vi "8X(json).vi"(0 "xml path":path=path "D:/wmgxml.xml", 1 "type":T4(ring)=enum."QSFP28", 5 "txtPath":path, 7 "singleItemInfo":T3[](array[typedef]), 9 "xml_detail":T1, 11 "TDD":T2) -> ()   [LabVIEW 2011]
uses:
  dataType/sSpec.ctl
  dataType/TDD.ctl
  dataType/xml_detail.ctl
panel:
  out "cycle item names":string[](array[string])
  out "midVar_time":string[](array[string])
  out "cycle items":string[](array[string])
  out "Terminat Points":dbl[](array[numeric])
  out "TDD spec cable":string
  out "TDD spec terminal":string
  out "Cable Points":dbl[](array[numeric])
  out "TestResult":string
  out "input_array_time":string[](array[string])
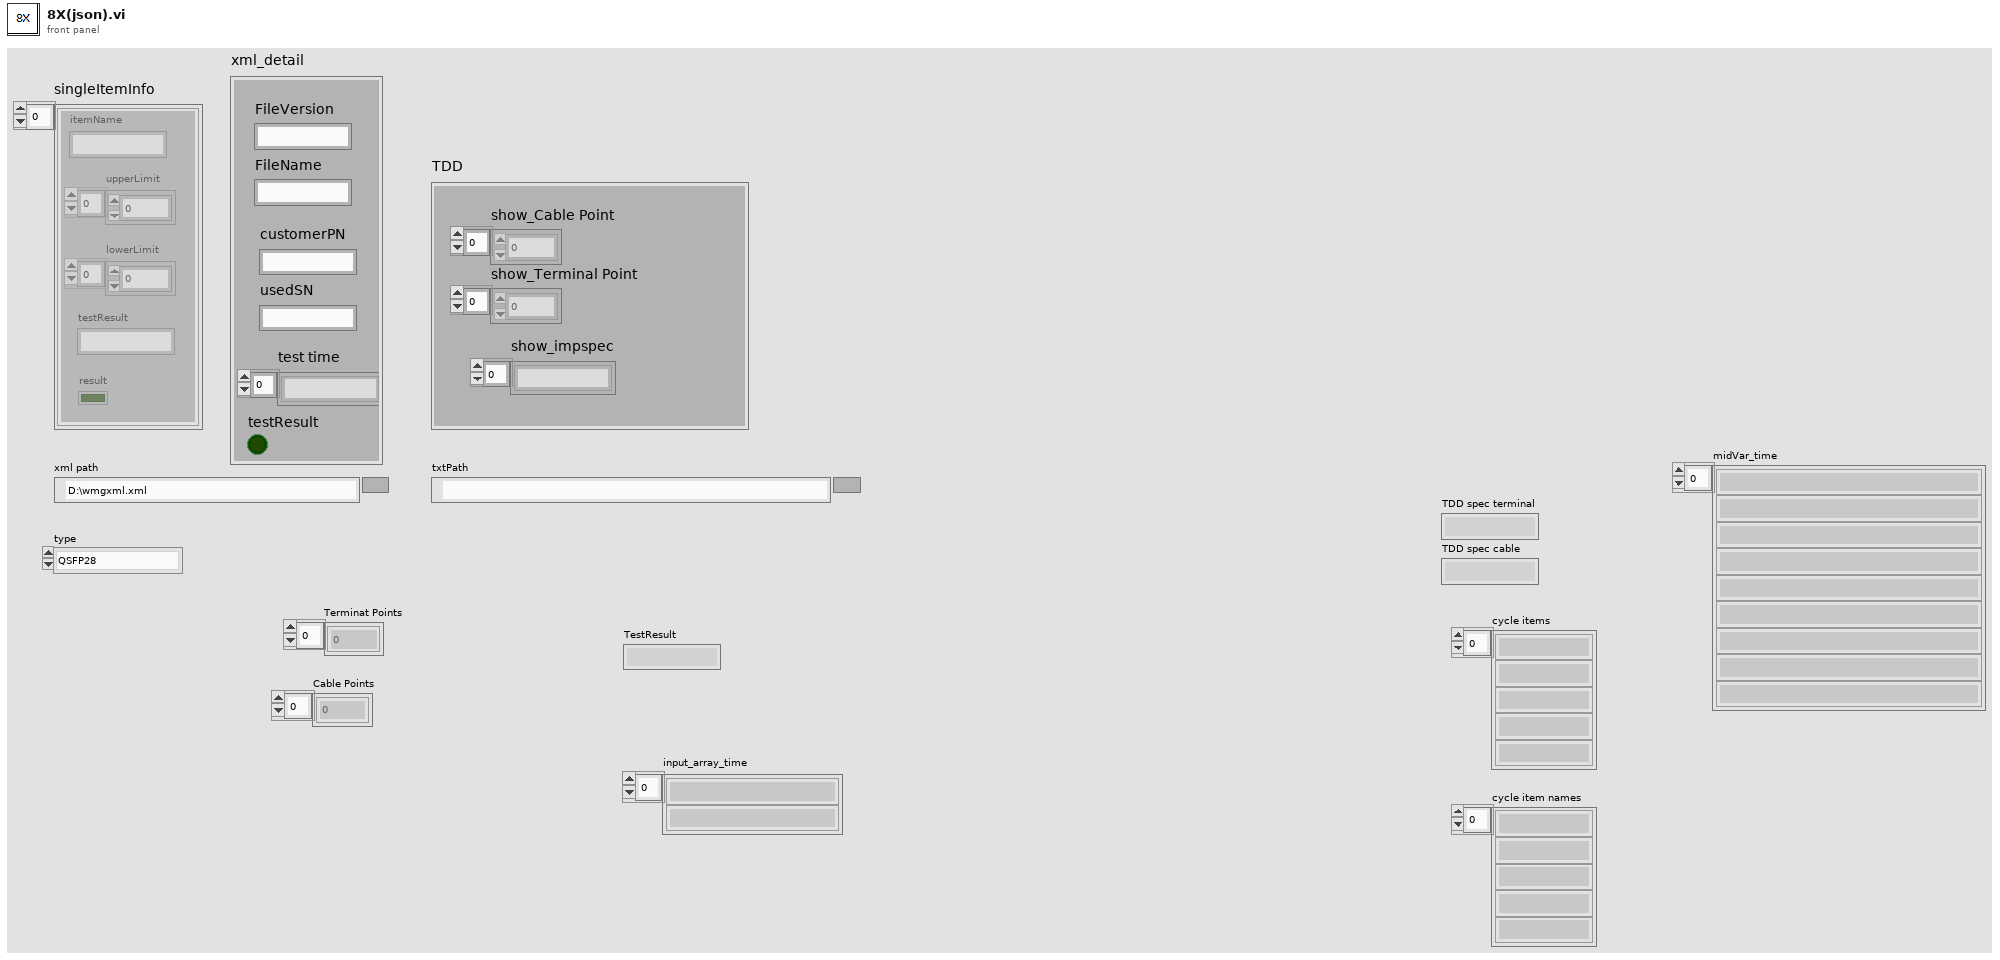
[diagram p1: front panel]
types:
  T1 = typedef "xml_detail.ctl" = cluster{"FileVersion":string, "FileName":string, "customerPN":string, "usedSN":string, "test time":string[], "testResult":bool}
  T2 = typedef "TDD.ctl" = cluster{"show_Cable Point":dbl[], "show_Terminal Point":dbl[], "show_impspec":string[]}
  T3 = typedef "sSpec.ctl" = cluster{"itemName":string, "upperLimit":dbl[], "lowerLimit":dbl[], "testResult":string, "result":bool}
  T4 = enum16{"MINI SAS HD 4X", "MINI SAS 4X", "SFP28", "QSFP28", "SFP+", "SLIM"}
  T5 = enum16{"open", "replace", "create", "open or create", "replace or create", "replace or create with confirmation"}
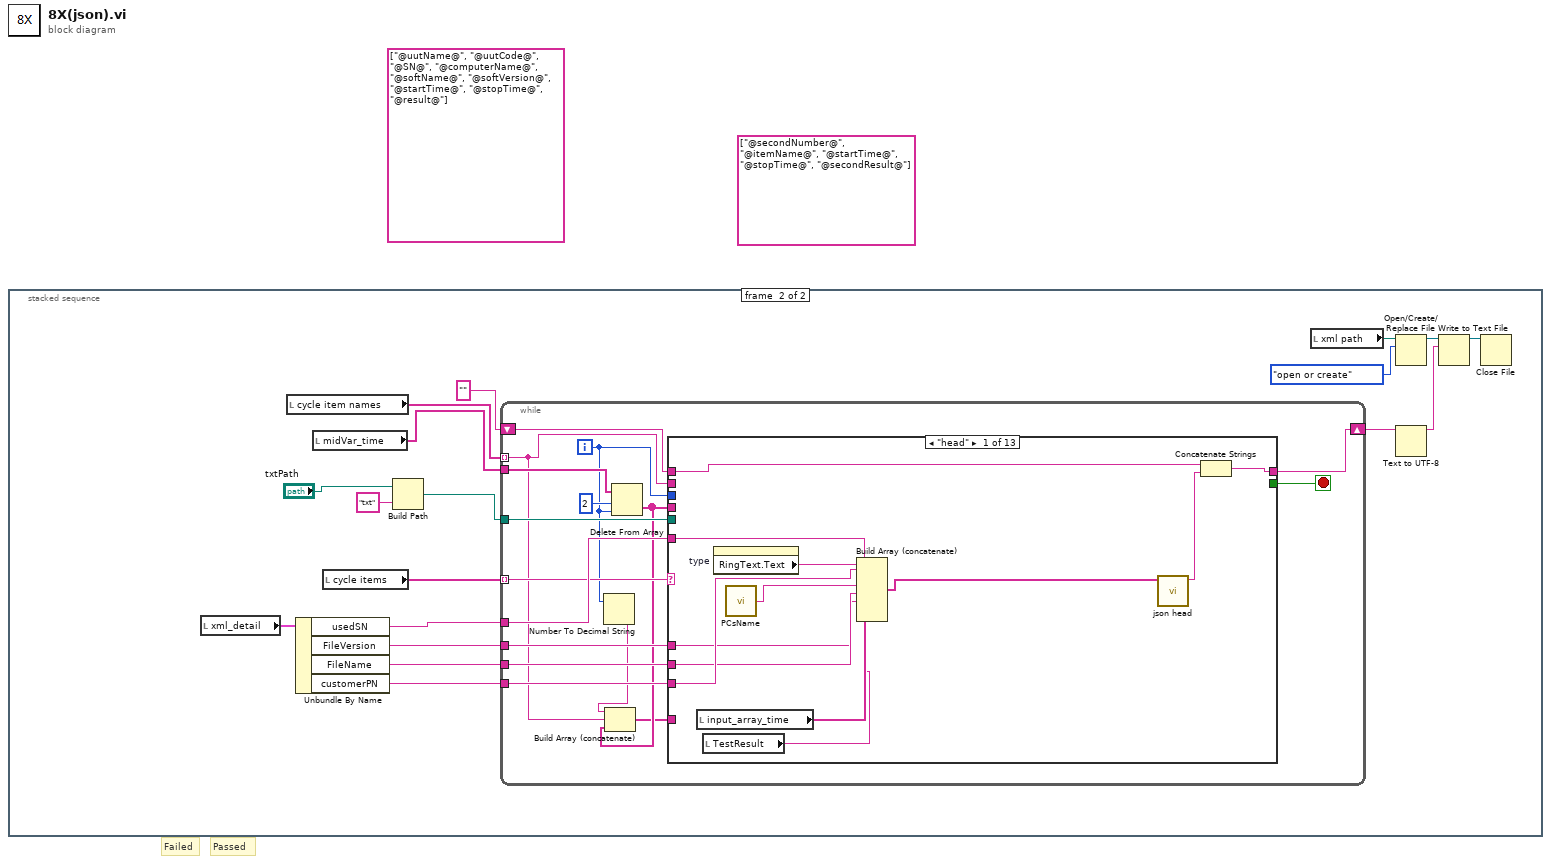
[diagram p0: block diagram]
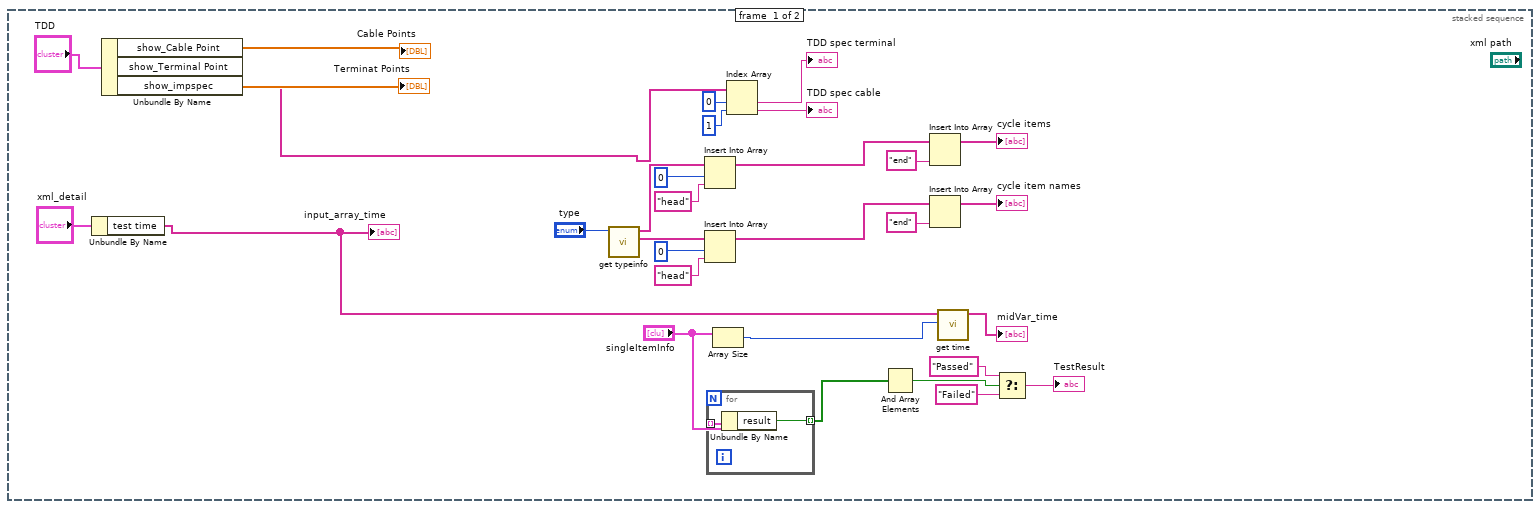
[diagram p2: hidden frame]
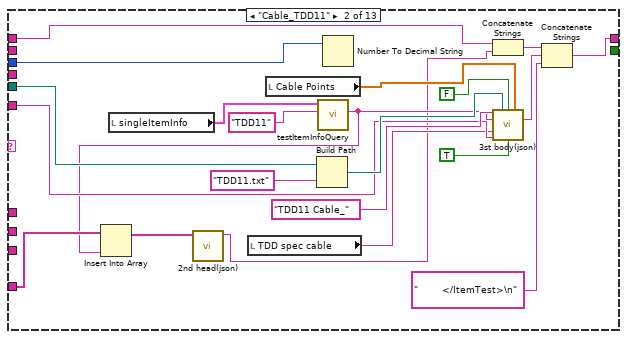
[diagram p3: hidden frame]
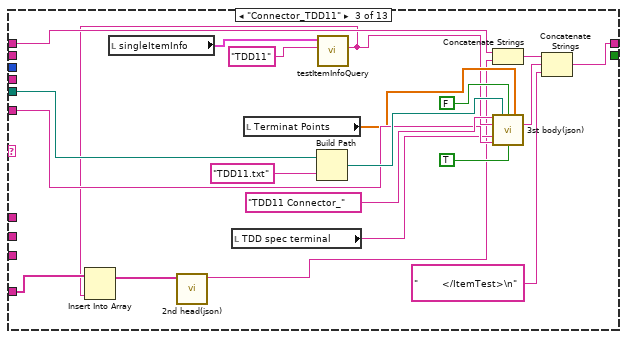
[diagram p4: hidden frame]
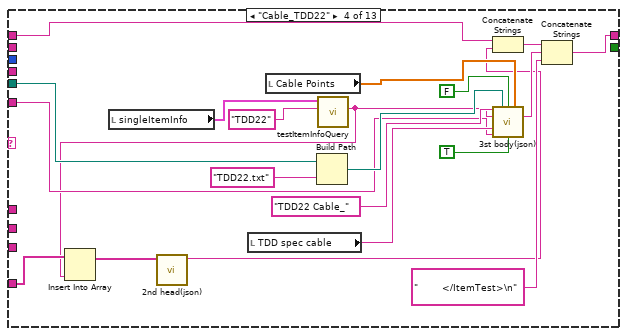
[diagram p5: hidden frame]
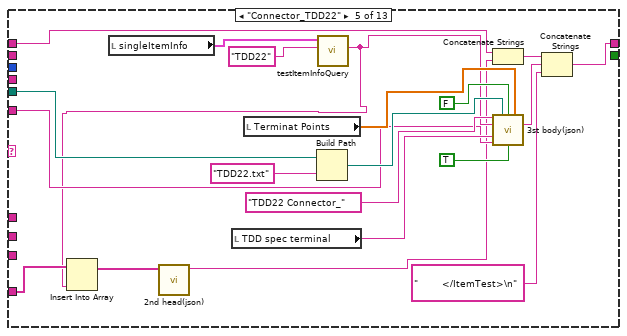
[diagram p6: hidden frame]
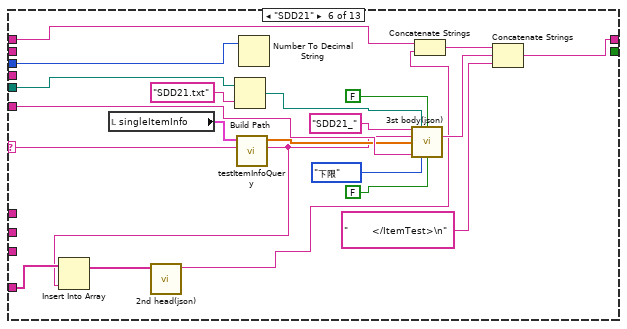
[diagram p7: hidden frame]
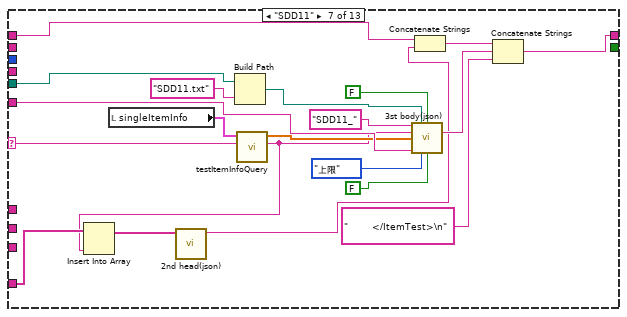
[diagram p8: hidden frame]
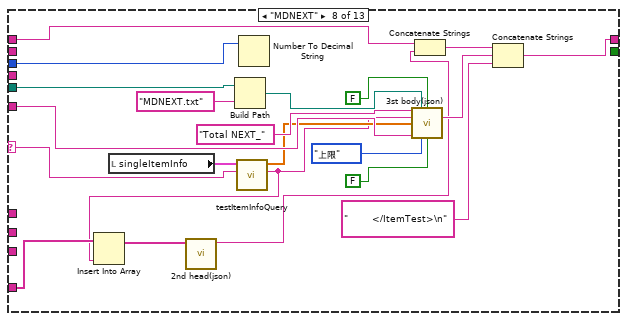
[diagram p9: hidden frame]
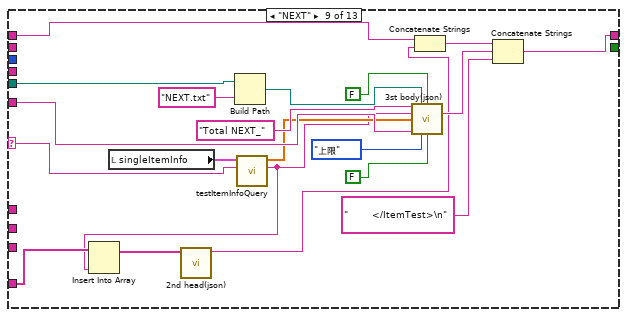
[diagram p10: hidden frame]
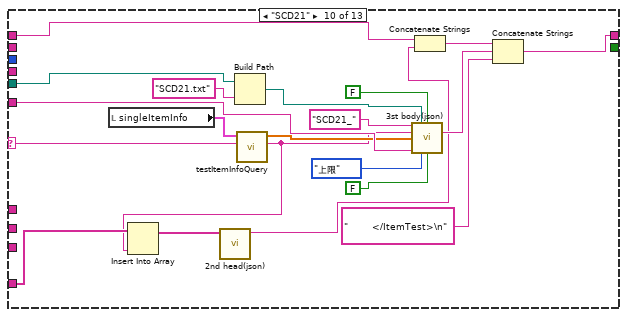
[diagram p11: hidden frame]
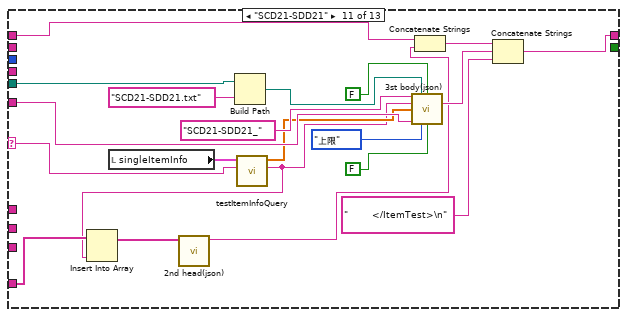
[diagram p12: hidden frame]
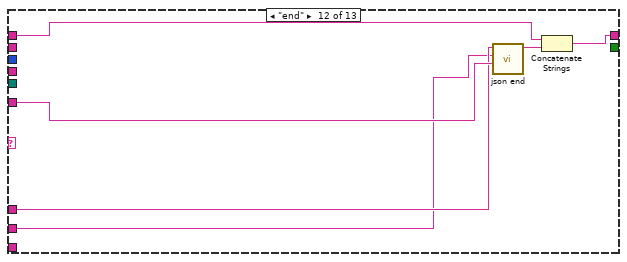
[diagram p13: hidden frame]
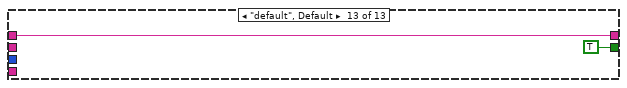
[diagram p14: hidden frame]
diagram:
  (unwired) string[] ["@uutName@", "@uutCode@", "@SN@", "@computerName@", "@softName@", "@softVersion@", "@startTime@", "@stopTime@", "@result@"]
  (unwired) string[] ["@secondNumber@", "@itemName@", "@startTime@", "@stopTime@", "@secondResult@"]
  # "Failed"
  # "Passed"
  n1 = stacked-sequence {
    frame #0 {
      n2 = Unbundle By Name("xml_detail") -> ("test time"=w1:string[])
      "input_array_time" <- w1
      n3 = Unbundle By Name("TDD") -> ("show_Cable Point"=→"Cable Points":dbl[], "show_Terminal Point"=→"Terminat Points":dbl[], "show_impspec"=w3:string[])
      n4 = call "get typeinfo.vi"("type"="type") -> ("second item names"=w15:string[], "test items"=w16:string[])  [unwired: 9 in]
      n5 = Insert Into Array(array=w16, index=0 ("索引"), new element="head" ("新元素/子数组")) -> (w25:string[])
      n6 = Insert Into Array(array=w15, index=0 ("索引"), new element="head" ("新元素/子数组")) -> (w19:string[])
      n7 = for {
        tunnel: "singleItemInfo" -> [w33] mode=indexing
        tunnel: [w32] -> w7 mode=indexing
        n8 = Unbundle By Name(w33) -> ("result"=w32:bool)
      }
      n9 = Array Size(array="singleItemInfo") -> (size(s)=w9:i32)
      n10 = Index Array(array=w3, index #1=0 ("索引"), index #2=1 ("索引")) -> (element #1=→"TDD spec terminal":string, element #2=→"TDD spec cable":string)
      n11 = And Array Elements(Boolean array=w7) -> (logical AND=w11:bool)
      n12 = Insert Into Array(array=w25, new element="end" ("新元素/子数组")) -> (→"cycle items":string[])  [unwired: 1 in]
      n13 = Insert Into Array(array=w19, new element="end" ("新元素/子数组")) -> (→"cycle item names":string[])  [unwired: 1 in]
      n14 = call "get time.vi"("item count"=w9, "input_array_time"=w1) -> ("midVar_time"=→"midVar_time":string[])  [unwired: 9 in]
      n15 = Select(t="Passed", s=w11, f="Failed") -> (s? t:f=→"TestResult":string)
    }
    frame #1 {
      n16 = local read "xml_detail"() -> (w38:T1)
      n17 = local read "cycle item names"() -> (w42:string[])
      n18 = Unbundle By Name(w38) -> ("usedSN"=w37:string, "FileVersion"=w36:string, "FileName"=w35:string, "customerPN"=w34:string)
      n19 = local read "midVar_time"() -> (w43:string[])
      n20 = local read "cycle items"() -> (w50:string[])
      n21 = Build Path(base path="txtPath", name or relative path="txt" ("名称或相对路径")) -> (appended path=w39:path)
      n22 = while {
        tunnel: w50 -> [w62] mode=indexing
        shift-right: [w66] -> w45
        shift-left: "" -> [w67]
        tunnel: w39 -> [w65]
        tunnel: w37 -> [w64]
        tunnel: w43 -> [w61]
        tunnel: w42 -> [w54] mode=indexing
        tunnel: w36 -> [w59]
        tunnel: w35 -> [w58]
        tunnel: w34 -> [w57]
        i -> [w56]
        stop <- w63 stop-if-true
        n23 = Number To Decimal String(number=w56) -> (decimal integer string=w55:string)  [unwired: 1 in]
        n24 = Delete From Array(array=w61, length=2 ("长度"), index=w56) -> (deleted portion=w53:string[])  [unwired: 1 out]
        n25 = Build Array (concatenate)(w55, w54, w53) -> (w52:string[])
        n26 = case shown="\"head\"" w62 {
          selector: w62 -> [_ _ _ _ _ w165 w186 w206 w227 w247 w267 _ _]
          tunnel: w67 -> [w79 w99 w120 w140 w160 w180 w201 w221 w242 w262 w282 w287 w290]
          tunnel: [w78 w96 w117 w137 w157 w177 w198 w218 w239 w259 w279 w286 w290] -> w66
          tunnel: w56 -> [_ w100 _ _ _ w181 _ w222 _ _ _ _ _]
          tunnel: w65 -> [_ w93 w114 w134 w154 w174 w195 w215 w236 w256 w276 _ _]
          tunnel: w64 -> [w74 w88 w109 w127 w147 w169 w190 w210 w231 w251 w271 w285 _]
          tunnel: [_ _ _ _ _ _ _ _ _ _ _ _ TRUE] -> w63
          tunnel: w53 -> [_ _ _ _ _ _ _ _ _ _ _ _ _]
          tunnel: w54 -> [_ _ _ _ _ _ _ _ _ _ _ _ _]
          tunnel: w59 -> [w71 _ _ _ _ _ _ _ _ _ _ w284 _]
          tunnel: w58 -> [w72 _ _ _ _ _ _ _ _ _ _ w283 _]
          tunnel: w57 -> [w75 _ _ _ _ _ _ _ _ _ _ _ _]
          tunnel: w52 -> [_ w83 w103 w123 w143 w163 w184 w204 w225 w245 w265 _ _]
          frame "head" {
            n27 = local read "input_array_time"() -> (w70:string[])
            n28 = local read "TestResult"() -> (w69:string)
            n29 = property on="type" class="Enum (严格)"() -> ("RingText.Text"=w76:string)  [unwired: 2 in, 2 out]
            n30 = call "PCsName.vi"() -> ("Computer Name"=w73:string)
            n31 = Build Array (concatenate)(w76, w75, w74, w73, w72, w71, w70, w69) -> (w68:string[])
            n32 = call "json head.vi"("information"=w68) -> ("midVar_Content"=w77:string)  [unwired: 10 in]
            n33 = Concatenate Strings(w79, w77) -> (w78:string)
          }
          frame "Cable_TDD11" {
            n34 = local read "singleItemInfo"() -> (w85:T3[])
            n35 = local read "TDD spec cable"() -> (w87:string)
            n36 = local read "Cable Points"() -> (w86:dbl[])
            n37 = Build Path(base path=w93, name or relative path="TDD11.txt" ("名称或相对路径")) -> (appended path=w91:path)
            n38 = call "testItemInfoQuery.vi"("testItem"="TDD11" ("test item"), "singleItemInfo"=w85) -> ("testResult"=w81:string)  [unwired: 8 in, 1 out]
            n39 = Insert Into Array(array=w83, new element=w81) -> (w82:string[])  [unwired: 1 in]
            n40 = call "2nd head(json).vi"("value"=w82) -> ("midVar_Content"=w80:string)  [unwired: 10 in]
            n41 = Number To Decimal String(number=w100) -> ()  [unwired: 1 in, 1 out]
            n42 = Concatenate Strings(w99, w80) -> (w97:string)
            n43 = call "3st body(json).vi"("third test item name"="TDD11 Cable_", "file path (dialog if empty)"=w91, "ABS?"=FALSE, "Points"=w86, "second result"=w81, "TDD spec"=w87, "SN"=w88, "TDD?"=TRUE) -> ("OutPutXml"=w95:string)  [unwired: 7 in]
            n44 = Concatenate Strings(w97, w95, "        </ItemTest>\n") -> (w96:string)
          }
          frame "Connector_TDD11" {
            n45 = local read "singleItemInfo"() -> (w106:T3[])
            n46 = local read "TDD spec terminal"() -> (w107:string)
            n47 = local read "Terminat Points"() -> (w108:dbl[])
            n48 = Build Path(base path=w114, name or relative path="TDD11.txt" ("名称或相对路径")) -> (appended path=w112:path)
            n49 = call "testItemInfoQuery.vi"("testItem"="TDD11" ("test item"), "singleItemInfo"=w106) -> ("testResult"=w102:string)  [unwired: 8 in, 1 out]
            n50 = Insert Into Array(array=w103, new element=w102) -> (w104:string[])  [unwired: 1 in]
            n51 = call "2nd head(json).vi"("value"=w104) -> ("midVar_Content"=w101:string)  [unwired: 10 in]
            n52 = Concatenate Strings(w120, w101) -> (w118:string)
            n53 = call "3st body(json).vi"("third test item name"="TDD11 Connector_", "file path (dialog if empty)"=w112, "ABS?"=FALSE, "Points"=w108, "second result"=w102, "TDD spec"=w107, "SN"=w109, "TDD?"=TRUE) -> ("OutPutXml"=w116:string)  [unwired: 7 in]
            n54 = Concatenate Strings(w118, w116, "        </ItemTest>\n") -> (w117:string)
          }
          frame "Cable_TDD22" {
            n55 = local read "singleItemInfo"() -> (w126:T3[])
            n56 = local read "TDD spec cable"() -> (w128:string)
            n57 = local read "Cable Points"() -> (w129:dbl[])
            n58 = Build Path(base path=w134, name or relative path="TDD22.txt" ("名称或相对路径")) -> (appended path=w132:path)
            n59 = call "testItemInfoQuery.vi"("testItem"="TDD22" ("test item"), "singleItemInfo"=w126) -> ("testResult"=w122:string)  [unwired: 8 in, 1 out]
            n60 = Insert Into Array(array=w123, new element=w122) -> (w124:string[])  [unwired: 1 in]
            n61 = call "2nd head(json).vi"("value"=w124) -> ("midVar_Content"=w121:string)  [unwired: 10 in]
            n62 = Concatenate Strings(w140, w121) -> (w138:string)
            n63 = call "3st body(json).vi"("third test item name"="TDD22 Cable_", "file path (dialog if empty)"=w132, "ABS?"=FALSE, "Points"=w129, "second result"=w122, "TDD spec"=w128, "SN"=w127, "TDD?"=TRUE) -> ("OutPutXml"=w136:string)  [unwired: 7 in]
            n64 = Concatenate Strings(w138, w136, "        </ItemTest>\n") -> (w137:string)
          }
          frame "Connector_TDD22" {
            n65 = local read "singleItemInfo"() -> (w146:T3[])
            n66 = local read "TDD spec terminal"() -> (w148:string)
            n67 = local read "Terminat Points"() -> (w149:dbl[])
            n68 = Build Path(base path=w154, name or relative path="TDD22.txt" ("名称或相对路径")) -> (appended path=w152:path)
            n69 = call "testItemInfoQuery.vi"("testItem"="TDD22" ("test item"), "singleItemInfo"=w146) -> ("testResult"=w142:string)  [unwired: 8 in, 1 out]
            n70 = Insert Into Array(array=w143, new element=w142) -> (w144:string[])  [unwired: 1 in]
            n71 = call "2nd head(json).vi"("value"=w144) -> ("midVar_Content"=w141:string)  [unwired: 10 in]
            n72 = Concatenate Strings(w160, w141) -> (w158:string)
            n73 = call "3st body(json).vi"("third test item name"="TDD22 Connector_", "file path (dialog if empty)"=w152, "ABS?"=FALSE, "Points"=w149, "second result"=w142, "TDD spec"=w148, "SN"=w147, "TDD?"=TRUE) -> ("OutPutXml"=w156:string)  [unwired: 7 in]
            n74 = Concatenate Strings(w158, w156, "        </ItemTest>\n") -> (w157:string)
          }
          frame "SDD21" {
            n75 = local read "singleItemInfo"() -> (w167:T3[])
            n76 = Build Path(base path=w174, name or relative path="SDD21.txt" ("名称或相对路径")) -> (appended path=w172:path)
            n77 = call "testItemInfoQuery.vi"("testItem"=w165, "singleItemInfo"=w167) -> ("testResult"=w162:string, "Limit"=w166:dbl[])  [unwired: 8 in]
            n78 = Insert Into Array(array=w163, new element=w162) -> (w164:string[])  [unwired: 1 in]
            n79 = call "2nd head(json).vi"("value"=w164) -> ("midVar_Content"=w161:string)  [unwired: 10 in]
            n80 = Number To Decimal String(number=w181) -> ()  [unwired: 1 in, 1 out]
            n81 = call "3st body(json).vi"("third test item name"="SDD21_", "file path (dialog if empty)"=w172, "ABS?"=FALSE, "second result"=w162, "single spec"=w166, "SN"=w169, "limit type"=enum16{"上限", "下限"}."下限", "TDD?"=FALSE) -> ("OutPutXml"=w176:string)  [unwired: 7 in]
            n82 = Concatenate Strings(w180, w161) -> (w178:string)
            n83 = Concatenate Strings(w178, w176, "        </ItemTest>\n") -> (w177:string)
          }
          frame "SDD11" {
            n84 = local read "singleItemInfo"() -> (w188:T3[])
            n85 = Build Path(base path=w195, name or relative path="SDD11.txt" ("名称或相对路径")) -> (appended path=w193:path)
            n86 = call "testItemInfoQuery.vi"("testItem"=w186, "singleItemInfo"=w188) -> ("testResult"=w183:string, "Limit"=w187:dbl[])  [unwired: 8 in]
            n87 = Insert Into Array(array=w184, new element=w183) -> (w185:string[])  [unwired: 1 in]
            n88 = call "2nd head(json).vi"("value"=w185) -> ("midVar_Content"=w182:string)  [unwired: 10 in]
            n89 = call "3st body(json).vi"("third test item name"="SDD11_", "file path (dialog if empty)"=w193, "ABS?"=FALSE, "second result"=w183, "single spec"=w187, "SN"=w190, "limit type"=enum16{"上限", "下限"}."上限", "TDD?"=FALSE) -> ("OutPutXml"=w197:string)  [unwired: 7 in]
            n90 = Concatenate Strings(w201, w182) -> (w199:string)
            n91 = Concatenate Strings(w199, w197, "        </ItemTest>\n") -> (w198:string)
          }
          frame "MDNEXT" {
            n92 = local read "singleItemInfo"() -> (w208:T3[])
            n93 = Build Path(base path=w215, name or relative path="MDNEXT.txt" ("名称或相对路径")) -> (appended path=w213:path)
            n94 = call "testItemInfoQuery.vi"("testItem"=w206, "singleItemInfo"=w208) -> ("testResult"=w203:string, "Limit"=w207:dbl[])  [unwired: 8 in]
            n95 = Insert Into Array(array=w204, new element=w203) -> (w205:string[])  [unwired: 1 in]
            n96 = call "2nd head(json).vi"("value"=w205) -> ("midVar_Content"=w202:string)  [unwired: 10 in]
            n97 = Number To Decimal String(number=w222) -> ()  [unwired: 1 in, 1 out]
            n98 = call "3st body(json).vi"("third test item name"="Total NEXT_", "file path (dialog if empty)"=w213, "ABS?"=FALSE, "second result"=w203, "single spec"=w207, "SN"=w210, "limit type"=enum16{"上限", "下限"}."上限", "TDD?"=FALSE) -> ("OutPutXml"=w217:string)  [unwired: 7 in]
            n99 = Concatenate Strings(w221, w202) -> (w219:string)
            n100 = Concatenate Strings(w219, w217, "        </ItemTest>\n") -> (w218:string)
          }
          frame "NEXT" {
            n101 = local read "singleItemInfo"() -> (w229:T3[])
            n102 = Build Path(base path=w236, name or relative path="NEXT.txt" ("名称或相对路径")) -> (appended path=w234:path)
            n103 = call "testItemInfoQuery.vi"("testItem"=w227, "singleItemInfo"=w229) -> ("testResult"=w224:string, "Limit"=w228:dbl[])  [unwired: 8 in]
            n104 = Insert Into Array(array=w225, new element=w224) -> (w226:string[])  [unwired: 1 in]
            n105 = call "2nd head(json).vi"("value"=w226) -> ("midVar_Content"=w223:string)  [unwired: 10 in]
            n106 = call "3st body(json).vi"("third test item name"="Total NEXT_", "file path (dialog if empty)"=w234, "ABS?"=FALSE, "second result"=w224, "single spec"=w228, "SN"=w231, "limit type"=enum16{"上限", "下限"}."上限", "TDD?"=FALSE) -> ("OutPutXml"=w238:string)  [unwired: 7 in]
            n107 = Concatenate Strings(w242, w223) -> (w240:string)
            n108 = Concatenate Strings(w240, w238, "        </ItemTest>\n") -> (w239:string)
          }
          frame "SCD21" {
            n109 = local read "singleItemInfo"() -> (w249:T3[])
            n110 = Build Path(base path=w256, name or relative path="SCD21.txt" ("名称或相对路径")) -> (appended path=w254:path)
            n111 = call "testItemInfoQuery.vi"("testItem"=w247, "singleItemInfo"=w249) -> ("testResult"=w244:string, "Limit"=w248:dbl[])  [unwired: 8 in]
            n112 = Insert Into Array(array=w245, new element=w244) -> (w246:string[])  [unwired: 1 in]
            n113 = call "2nd head(json).vi"("value"=w246) -> ("midVar_Content"=w243:string)  [unwired: 10 in]
            n114 = call "3st body(json).vi"("third test item name"="SCD21_", "file path (dialog if empty)"=w254, "ABS?"=FALSE, "second result"=w244, "single spec"=w248, "SN"=w251, "limit type"=enum16{"上限", "下限"}."上限", "TDD?"=FALSE) -> ("OutPutXml"=w258:string)  [unwired: 7 in]
            n115 = Concatenate Strings(w262, w243) -> (w260:string)
            n116 = Concatenate Strings(w260, w258, "        </ItemTest>\n") -> (w259:string)
          }
          frame "SCD21-SDD21" {
            n117 = local read "singleItemInfo"() -> (w269:T3[])
            n118 = Build Path(base path=w276, name or relative path="SCD21-SDD21.txt" ("名称或相对路径")) -> (appended path=w274:path)
            n119 = call "testItemInfoQuery.vi"("testItem"=w267, "singleItemInfo"=w269) -> ("testResult"=w264:string, "Limit"=w268:dbl[])  [unwired: 8 in]
            n120 = Insert Into Array(array=w265, new element=w264) -> (w266:string[])  [unwired: 1 in]
            n121 = call "2nd head(json).vi"("value"=w266) -> ("midVar_Content"=w263:string)  [unwired: 10 in]
            n122 = call "3st body(json).vi"("third test item name"="SCD21-SDD21_", "file path (dialog if empty)"=w274, "ABS?"=FALSE, "second result"=w264, "single spec"=w268, "SN"=w271, "limit type"=enum16{"上限", "下限"}."上限", "TDD?"=FALSE) -> ("OutPutXml"=w278:string)  [unwired: 7 in]
            n123 = Concatenate Strings(w282, w263) -> (w280:string)
            n124 = Concatenate Strings(w280, w278, "        </ItemTest>\n") -> (w279:string)
          }
          frame "end" {
            n125 = call "json end.vi"("SN"=w285, "FilePath"=w283, "FileVer"=w284) -> ("midVar_Content"=w288:string)  [unwired: 8 in]
            n126 = Concatenate Strings(w287, w288) -> (w286:string)
          }
          frame "default", Default {
          }
        }
      }
      n127 = local read "xml path"() -> (w44:path)
      n128 = Open/Create/Replace File(file path (use dialog)=w44, operation (0:open)=T5."open or create" ("操作(0:open)")) -> (refnum out=w48:refnum<file>)  [unwired: 4 in, 2 out]
      n129 = Text to UTF-8(11:w45) -> (3:w46:string)  [unwired: 1 in, 1 out]
      n130 = Write to Text File(file (use dialog)=w48, text=w46) -> (refnum out=w47:refnum<file>)  [unwired: 2 in, 2 out]
      n131 = Close File(refnum=w47) -> ()  [unwired: 1 in, 2 out]
    }
  }
